vi "Set Study CFG.vi"(8 "error in (no error)":errorcluster, 10 "Study CFG":string, 11 "Study Base in":refnum<class "Study Base.lvclass">) -> (0 "error out":errorcluster, 3 "Study Base out":refnum<class "Study Base.lvclass">)   [LabVIEW 2023, in "HAL GOOP4.lvlib" / "Study Base.lvclass"]
uses:
  Study Base.lvclass
  Study Base.lvclass/Study Base.ctl
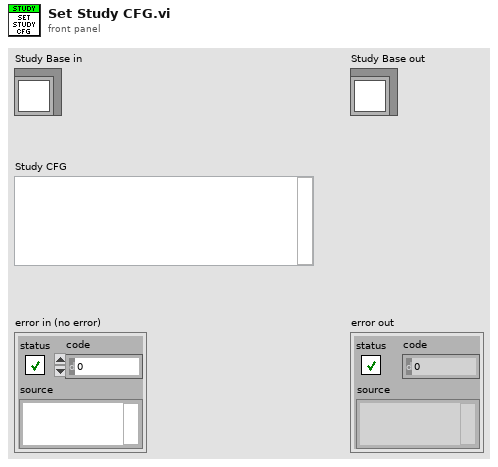
[diagram p1: front panel]
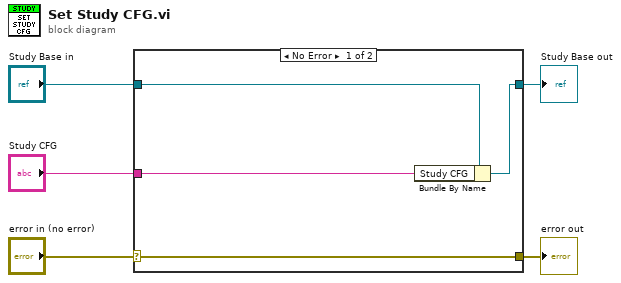
[diagram p0: block diagram]
diagram:
  n1 = case shown="No Error" "error in (no error)" {
    selector: "error in (no error)" -> [w9 w10]
    tunnel: [w9 w10] -> w4
    tunnel: [w7 w11] -> w2
    tunnel: "Study Base in" -> [w8 w11]
    tunnel: "Study CFG" -> [w6 _]
    frame No Error {
      n2 = Bundle By Name(cluster=w8, "Study CFG"=w6) -> (w7:refnum<class "Study Base.lvclass">)
    }
    frame Error {
    }
  }
  "error out" <- w4
  "Study Base out" <- w2
